vi "条件查找数组元素(1D VI-REF).vi"(8 "error in (no error)":errorcluster caption="错误输入（无错误）", 10 "条件数组":bool[](array[boolean]), 11 "输入数组":refnum<vi>[](array[refnum])) -> (0 "error out":errorcluster caption="错误输出", 2 "符合条件元素索引":i32[](array[numeric]), 3 "符合条件元素":refnum<vi>[](array[refnum]))   [LabVIEW 2011]
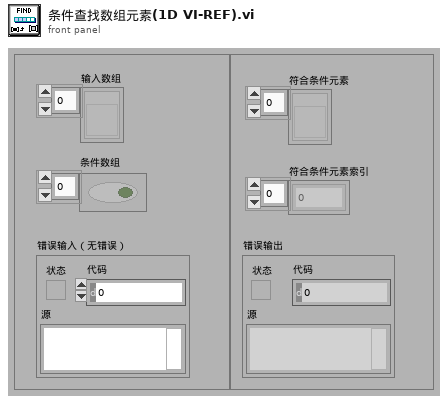
[diagram p1: front panel]
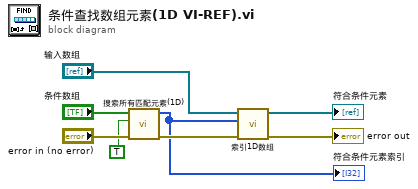
[diagram p0: block diagram]
diagram:
  n1 = call-poly "搜索所有匹配元素(1D).vi"("error in (no error)"="error in (no error)", "元素"=TRUE, "数组"="条件数组") -> ("error out"=w5:errorcluster, "匹配元素索引"=w1:i32[])  [unwired: 6 in, 1 out]
  "符合条件元素索引" <- w1
  n2 = call-poly "索引1D数组.vi"("error in (no error)"=w5, "索引"=w1, "输入数组"="输入数组") -> ("error out"=→"error out":errorcluster, "元素"=→"符合条件元素":refnum<vi>[])  [unwired: 7 in]
